vi "Untitled 13.vi"() -> ()   [LabVIEW 2025]
uses:
  PLC_Data_Config.ctl
  PLC_Data.ctl
  PLC_Data_Type.ctl
  PLC_Module.lvclass/PLC_Module.ctl
  PLC_Module.lvclass
  <vilib>/addons/Tools/Unicode/UTF8 Tools.lvlib
panel:
  out "Configuration":T1
  out "data":T4
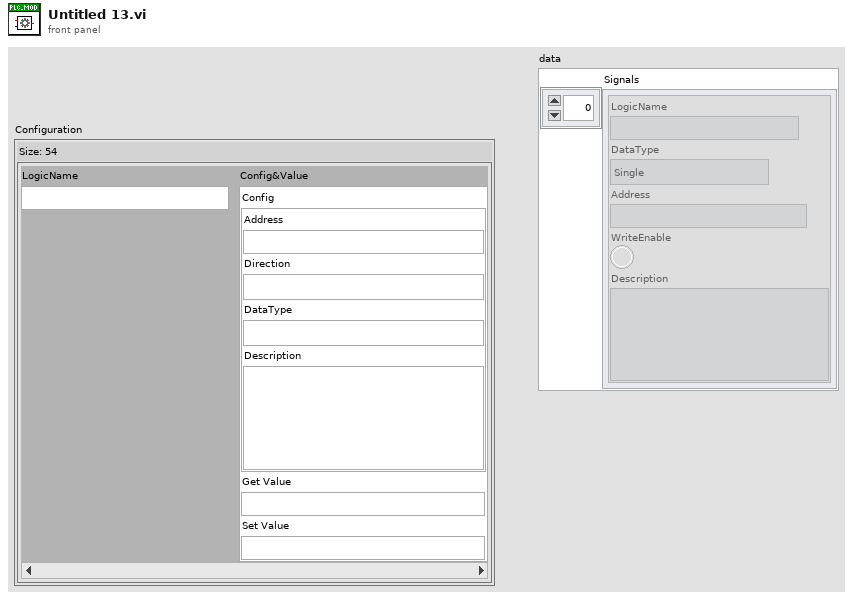
[diagram p1: front panel]
types:
  T1 = typedef "PLC_Module.lvlib/PLC_Module.lvclass/PLC_Data_Config.ctl" = map{string, cluster{"Config":T2, "Get Value":string, "Set Value":string}}
  T2 = typedef "PLC_Module.lvlib/PLC_Module.lvclass/PLC_Data.ctl" = cluster{"Address":string, "Direction":enum16{"PC->PLC", "PLC->PC"}, "DataType":T3, "Description":string}
  T3 = typedef "PLC_Module.lvlib/PLC_Module.lvclass/PLC_Data_Type.ctl" = enum16{"Boolean", "Single Float", "U8", "U32", "U32_Array", "String"}
  T4 = cluster{"Signals":cluster{"LogicName":string, "DataType":enum16{"Single", "Double", "I8", "I16", "I32", "I64", "U8", "U16", "U32", "U64", "Boolean", "String", "U8Array"}, "Address":string, "WriteEnable":bool, "Description":string}[]}
  T5 = cluster{"LogicName":string, "DataType":enum16{"Single", "Double", "I8", "I16", "I32", "I64", "U8", "U16", "U32", "U64", "Boolean", "String", "U8Array"}, "Address":string, "WriteEnable":bool, "Description":string}[]
  T6 = cluster{"Config":T2, "Get Value":string, "Set Value":string}
  T7 = enum16{"Single", "Double", "I8", "I16", "I32", "I64", "U8", "U16", "U32", "U64", "Boolean", "String", "U8Array"}
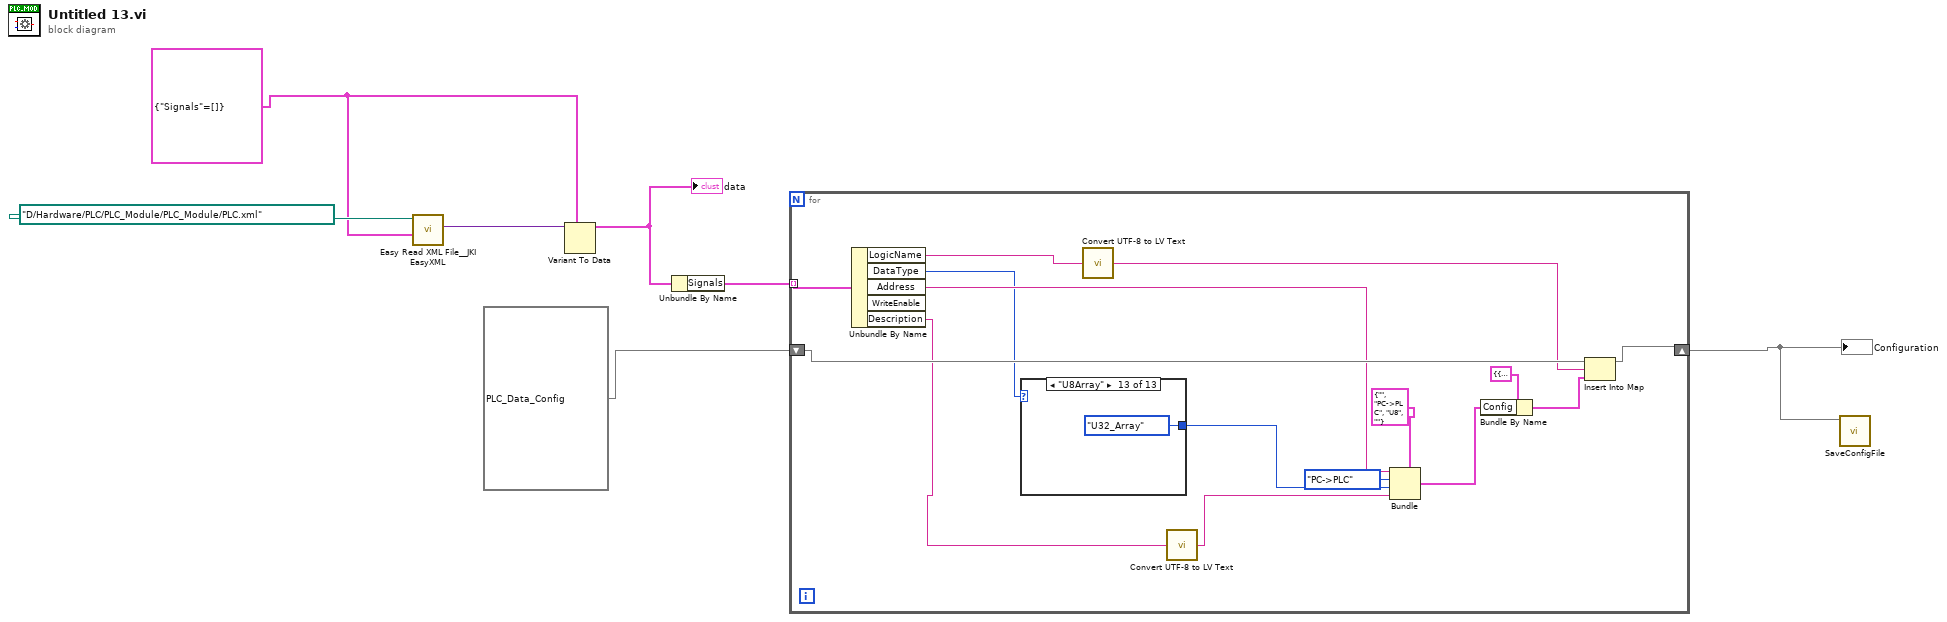
[diagram p0: block diagram]
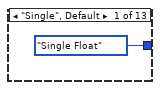
[diagram p2: hidden frame]
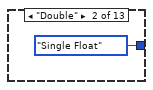
[diagram p3: hidden frame]
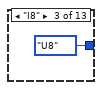
[diagram p4: hidden frame]
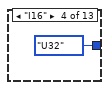
[diagram p5: hidden frame]
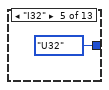
[diagram p6: hidden frame]
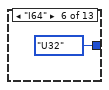
[diagram p7: hidden frame]
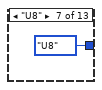
[diagram p8: hidden frame]
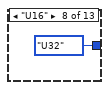
[diagram p9: hidden frame]
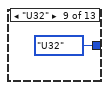
[diagram p10: hidden frame]
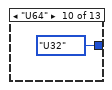
[diagram p11: hidden frame]
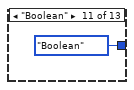
[diagram p12: hidden frame]
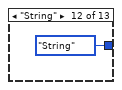
[diagram p13: hidden frame]
diagram:
  w5 = T4 {"Signals"=[]} ("Configuration")
  n1 = call <vilib>:"Easy Read XML File__JKI EasyXML.vi"("LabVIEW Data (Type)"=w5, "XML File Path"=path "D:/Hardware/PLC/PLC_Module/PLC_Module/PLC.xml") -> ("LabVIEW Data"=w6:variant)  [unwired: 7 in, 2 out]
  n2 = Variant To Data(type=w5, Variant=w6) -> (data=w4:T4)  [unwired: 1 in, 1 out]
  "data" <- w4
  n3 = Unbundle By Name(w4) -> ("Signals"=w3:T5)
  n4 = for {
    tunnel: w3 -> [w21] mode=indexing
    shift-right: [w20] -> w1
    shift-left: T1 {} ("Configuration") -> [w22]
    n5 = Unbundle By Name(w21) -> ("LogicName"=w11:string, "DataType"=w13:T7, "Address"=w15:string, "Description"=w9:string)  [unwired: 1 out]
    n6 = case shown="\"U8Array\"" w13 {
      tunnel: [PLC_Data_Type."Single Float" ("DataType") PLC_Data_Type."Single Float" ("DataType") PLC_Data_Type."U8" ("DataType") PLC_Data_Type."U32" ("DataType") PLC_Data_Type."U32" ("DataType") PLC_Data_Type."U32" ("DataType") PLC_Data_Type."U8" ("DataType") PLC_Data_Type."U32" ("DataType") PLC_Data_Type."U32" ("DataType") PLC_Data_Type."U32" ("DataType") PLC_Data_Type."Boolean" ("DataType") PLC_Data_Type."String" ("DataType") PLC_Data_Type."U32_Array" ("DataType")] -> w12
      frame "Single", Default {
      }
      frame "Double" {
      }
      frame "I8" {
      }
      frame "I16" {
      }
      frame "I32" {
      }
      frame "I64" {
      }
      frame "U8" {
      }
      frame "U16" {
      }
      frame "U32" {
      }
      frame "U64" {
      }
      frame "Boolean" {
      }
      frame "String" {
      }
      frame "U8Array" {
      }
    }
    n7 = call <vilib>:"Convert UTF-8 to LV Text.vi"("UTF-8 Text"=w11) -> ("LV Text"=w10:string)  [unwired: 13 in, 1 out]
    n8 = call <vilib>:"Convert UTF-8 to LV Text.vi"("UTF-8 Text"=w9) -> ("LV Text"=w8:string)  [unwired: 13 in, 1 out]
    n9 = Bundle(cluster=T2 {"Address"="", "Direction"=enum."PC->PLC", "DataType"=enum."U8", "Description"=""} ("Config"), "Address"=w15, "Direction"=enum16{"PC->PLC", "PLC->PC"}."PC->PLC", "DataType"=w12, "Description"=w8) -> (w16:T2)
    n10 = Bundle By Name(cluster=T6 {"Config"={"Address"="", "Direction"=enum."PC->PLC", "DataType"=enum."Boolean", "Description"=""}, "Get Value"="", "Set Value"=""} ("value"), "Config"=w16) -> (w18:T6)
    n11 = Insert Into Map(map in=w22, key=w10, value=w18) -> (map out=w20:T1)  [unwired: 2 out]
  }
  "Configuration" <- w1
  n12 = call "SaveConfigFile.vi"("Configuration"=w1) -> ()  [unwired: 10 in, 1 out]
